vi "AssertsSubpanelExecStateBad.vi"(0 "VI Reference In":refnum<vi>, 1 "Label (VI Title)":string="Default", 11 "error in":errorcluster) -> (4 "VI Reference Out":refnum<vi>, 15 "error out":errorcluster)   [LabVIEW 2016, in "DronaTest.lvlib"]
uses:
  APIs/Stimulus/ControlValue/ValueSignalByPathString.vi
  APIs/Assert/AssertSubpanel/AssertSubpanelVIExecBad.vi
  <vilib>/addons/_JKI Toolkits/Caraya/classes/Assert/Assert Error.vi
  DronaTest.lvlib
  <vilib>/addons/_JKI Toolkits/Caraya/classes/Test/Test.lvclass
  Drona.lvlib
  APIs/Stimulus/ControlValue/ControlValue.lvlib
  <vilib>/addons/_JKI Toolkits/Caraya/classes/Assert/Assert.lvclass
  APIs/Assert/AssertSubpanel/AssertSubpanel.lvlib
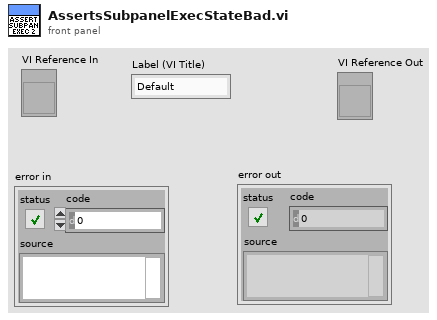
[diagram p1: front panel]
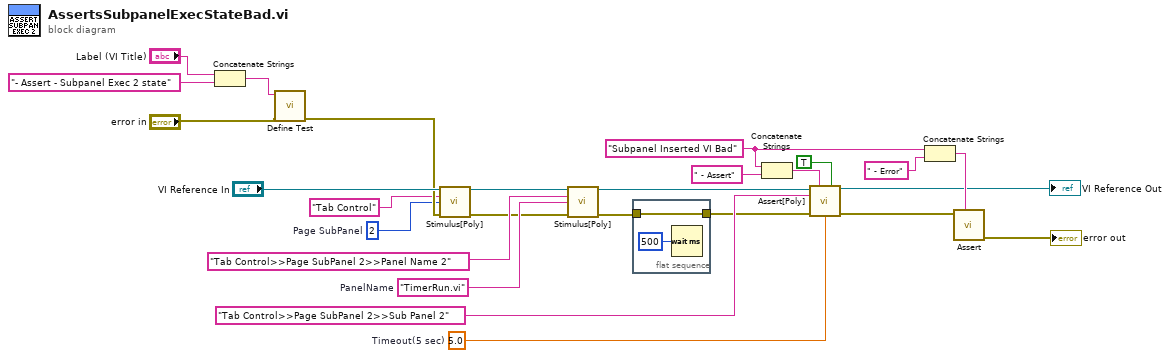
[diagram p0: block diagram]
diagram:
  w5 = 2  # Page SubPanel
  w11 = "TimerRun.vi"  # PanelName
  w18 = "Subpanel Inserted VI Bad" ("Label")
  w14 = 5.0  # Timeout(5 sec)
  n1 = Concatenate Strings("Label (VI Title)", "- Assert - Subpanel Exec 2 state" ("string")) -> (w22:string)
  n2 = call <vilib>:"Define Test.vi"("error in (no error)"="error in", "Label (VI Title)"=w22) -> ("error out"=w7:errorcluster)  [unwired: 9 in]
  n3 = call-poly "Stimulus[Poly].vi"("VI Reference In"="VI Reference In", "Control Path"="Tab Control", "Value (Signaling)"=w5, "error in"=w7) -> ("VI Reference Out"=w8:refnum<vi>, "error out"=w4:errorcluster)  [unwired: 10 in]
  n4 = call-poly "Stimulus[Poly].vi"("VI Reference In"=w8, "Control Path"="Tab Control>>Page SubPanel 2>>Panel Name 2", "Value (Signaling)"=w11, "error in"=w4) -> ("VI Reference Out"=w2:refnum<vi>, "error out"=w10:errorcluster)  [unwired: 10 in]
  n5 = flat-sequence {
    tunnel: w10 -> [w28]
    tunnel: [w28] -> w3
    frame #0 {
      n6 = Wait (ms)(milliseconds to wait=u32 500) -> ()  [unwired: 1 out]
    }
  }
  n7 = Concatenate Strings(w18, " - Assert" ("string")) -> (w16:string)
  n8 = call-poly "Assert[Poly].vi"("VI Reference In"=w2, "Test Label"=w16, "Assert Only? (F)"=TRUE, "Control Path"="Tab Control>>Page SubPanel 2>>Sub Panel 2", "Error In"=w3, "Timeout(5 sec)"=w14) -> ("VI Reference Out"=→"VI Reference Out":refnum<vi>, "Error Out"=w12:errorcluster)  [unwired: 8 in]
  n9 = Concatenate Strings(w18, " - Error" ("string")) -> (w26:string)
  n10 = call-poly <vilib>:"Assert.vi"("Label"=w26, "Error?"=w12) -> ("error out"=→"error out":errorcluster)  [unwired: 9 in]
